vi "Get Clock (Calendar).vi"(0 "VISA resource name":refnum<visa-resource-name>, 11 "error in (no error)":errorcluster) -> (3 "Hour":i32, 4 "VISA resource name out":refnum<visa-resource-name>, 6 "Minute":i32, 8 "Second":i32, 10 "Day":i32, 13 "Year":i32, 14 "Month":i32, 15 "error out":errorcluster)   [LabVIEW 2014, in "Fluke 5XXX Series Multicalibrators.lvlib"]
doc: "This VI returns the instrument's internal clock and calendar settings.\n\nNote:\n\nThis VI is available only for instrument models 5520A, 5700A, 5720A and 57LFC."
uses:
  Fluke 5XXX Series Multicalibrators.lvlib
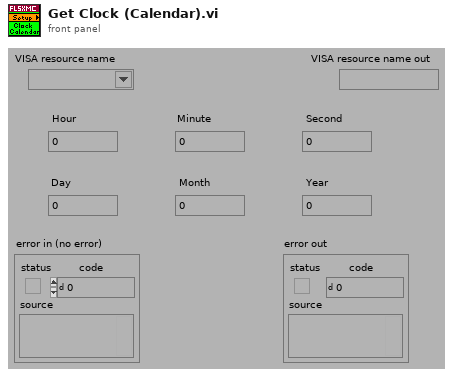
[diagram p1: front panel]
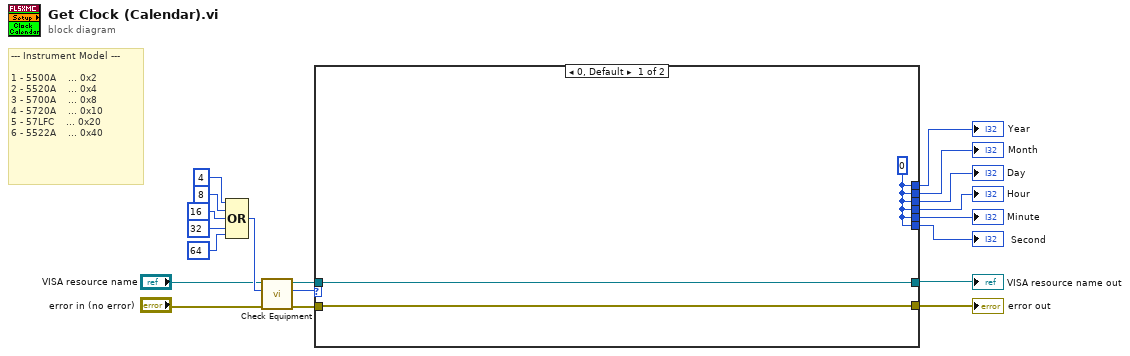
[diagram p0: block diagram]
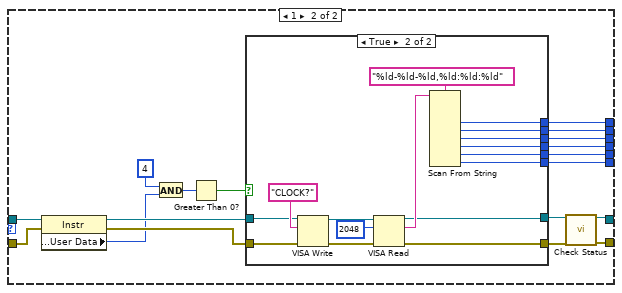
[diagram p2: hidden frame]
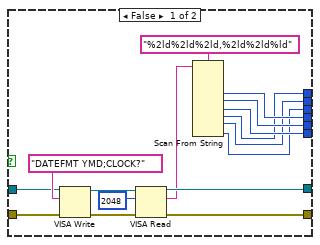
[diagram p3: hidden frame]
diagram:
  # "--- Instrument Model ---\n\n1 - 5500A    ... 0x2\n2 - 5520A    ... 0x4\n3 - 5700A    ... 0x8\n4 - 5720A    ... 0x10\n5 - 57LFC    ... 0x20\n6 - 5522A    ... 0x40"
  n1 = Compound Arithmetic op=OR(4 ("Numeric"), 8 ("Numeric"), 16 ("Numeric"), 32 ("Numeric"), 64 ("Numeric")) -> (w13:i32)
  n2 = call "Check Equipment.vi"("error in (no error)"="error in (no error)", "Bit Mask"=w13, "VISA resource name"="VISA resource name") -> ("error out"=w16:errorcluster, "Present?"=w14:u32, "VISA resource name out"=w15:refnum<visa-resource-name>)  [unwired: 6 in]
  n3 = case shown="0, Default" w14 {
    tunnel: [w21 w39] -> w12
    tunnel: w16 -> [w22 w29]
    tunnel: w15 -> [w21 w30]
    tunnel: [w22 w40] -> w11
    tunnel: [w20 w36] -> w8
    tunnel: [w20 w35] -> w7
    tunnel: [w20 w34] -> w6
    tunnel: [w20 w33] -> w5
    tunnel: [w20 w32] -> w4
    tunnel: [w20 w31] -> w3
    frame 0, Default {
      w20 = 0
    }
    frame 1 {
      n4 = property class="Instr"(reference=w30, error in=w29) -> (reference out=w28:refnum<visa-resource-name>, error out=w27:errorcluster, "General Settings:User Data"=w26:u32)
      n5 = And(x=u32 4 ("Numeric"), y=w26) -> (x .and. y?=w24:u32)
      n6 = Greater Than 0?(x=w24) -> (x > 0?=w23:bool)
      n7 = case shown="True" w23 {
        tunnel: w27 -> [w48 w66]
        tunnel: [w51 w65] -> w38
        tunnel: [w50 w64] -> w37
        tunnel: w28 -> [w49 w63]
        tunnel: [w44 w62] -> w36
        tunnel: [w43 w61] -> w35
        tunnel: [w42 w60] -> w34
        tunnel: [w47 w59] -> w33
        tunnel: [w46 w58] -> w32
        tunnel: [w45 w57] -> w31
        frame False {
          n8 = VISA Write(VISA resource name=w49, write buffer="DATEFMT YMD;CLOCK?", error in (no error)=w48) -> (VISA resource name out=w54:refnum<visa-resource-name>, error out=w53:errorcluster)  [unwired: 1 out]
          n9 = VISA Read(VISA resource name=w54, byte count=u32 2048 ("byte count (0)"), error in (no error)=w53) -> (VISA resource name out=w50:refnum<visa-resource-name>, read buffer=w41:string, error out=w51:errorcluster)  [unwired: 1 out]
          n10 = Scan From String(format string="%2ld%2ld%2ld,%2ld%2ld%ld", input string=w41) -> (output 1=w47:i32, output 2=w46:i32, output 3=w45:i32, output 4=w44:i32, output 5=w43:i32, output 6=w42:i32)  [unwired: 8 in, 3 out]
        }
        frame True {
          n11 = VISA Write(VISA resource name=w63, write buffer="CLOCK?", error in (no error)=w66) -> (VISA resource name out=w70:refnum<visa-resource-name>, error out=w69:errorcluster)  [unwired: 1 out]
          n12 = VISA Read(VISA resource name=w70, byte count=u32 2048 ("byte count (0)"), error in (no error)=w69) -> (VISA resource name out=w64:refnum<visa-resource-name>, read buffer=w67:string, error out=w65:errorcluster)  [unwired: 1 out]
          n13 = Scan From String(format string="%ld-%ld-%ld,%ld:%ld:%ld", input string=w67) -> (output 1=w62:i32, output 2=w61:i32, output 3=w60:i32, output 4=w59:i32, output 5=w58:i32, output 6=w57:i32)  [unwired: 8 in, 3 out]
        }
      }
      n14 = call "Check Status.vi"("VISA resource name"=w37, "error in (no error)"=w38) -> ("VISA resource name out"=w39:refnum<visa-resource-name>, "error out"=w40:errorcluster)  [unwired: 12 in]
    }
  }
  "Hour" <- w5
  "Minute" <- w4
  "Second" <- w3
  "Day" <- w6
  "Month" <- w7
  "Year" <- w8
  "VISA resource name out" <- w12
  "error out" <- w11
